vi "TWM Client Cmd Stop.vi"(5 "timeout [ms] (3000)":i32=3000, 7 "end of packet key":string="TWM:command:EndOfPacket", 8 "error in":errorcluster, 11 "handle":i32) -> (0 "error out":errorcluster, 3 "handle out":i32)   [LabVIEW 2020, in "TWM Client.lvlib"]
doc: "Write Stop command packet to TWM server. It will stop the measurement."
uses:
  TWM Client.lvlib
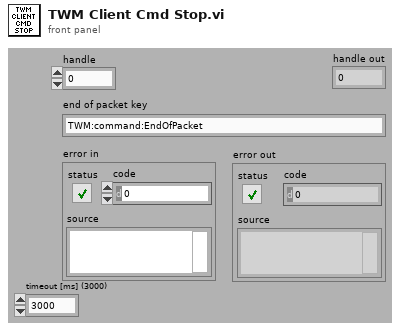
[diagram p1: front panel]
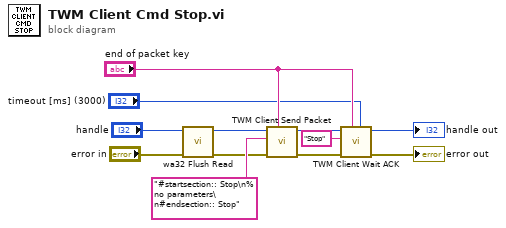
[diagram p0: block diagram]
diagram:
  n1 = call "wa32 Flush Read.vi"("error in"="error in", "handle"="handle") -> ("error out"=w3:errorcluster, "handle out"=w2:i32)  [unwired: 7 in, 1 out]
  n2 = call "TWM Client Send Packet.vi"("end of packet key"="end of packet key", "error in"=w3, "command string"="#startsection:: Stop\n% no parameters\n#endsection:: Stop", "handle"=w2) -> ("error out"=w11:errorcluster, "handle out"=w8:i32)  [unwired: 6 in]
  n3 = call "TWM Client Wait ACK.vi"("timeout [ms] (3000)"="timeout [ms] (3000)", "key string"="end of packet key", "error in"=w11, "command header"="Stop", "handle"=w8) -> ("error out"=→"error out":errorcluster, "handle out"=→"handle out":i32)  [unwired: 5 in]
